vi "FTW-JSON-SetFlags-Encoding.vi"(0 "JSON Object":refnum<class "FTW-JSON.lvclass">, 5 "Indent Spaces":i32=4, 7 "Escape Unicode":bool=TRUE, 9 "Sort Keys":bool, 11 "error in":errorcluster, 12 "Floating Point Significant Digits":i32=16) -> (4 "JSON Object out":refnum<class "FTW-JSON.lvclass">, 15 "error out":errorcluster)   [LabVIEW 2013, in "FTW-JSON.lvclass"]
uses:
  FTW-JSON.lvclass
  FTW-JSON.lvclass/FTW-JSON.ctl
panel:
  # "Inputs"
  # "Outputs"
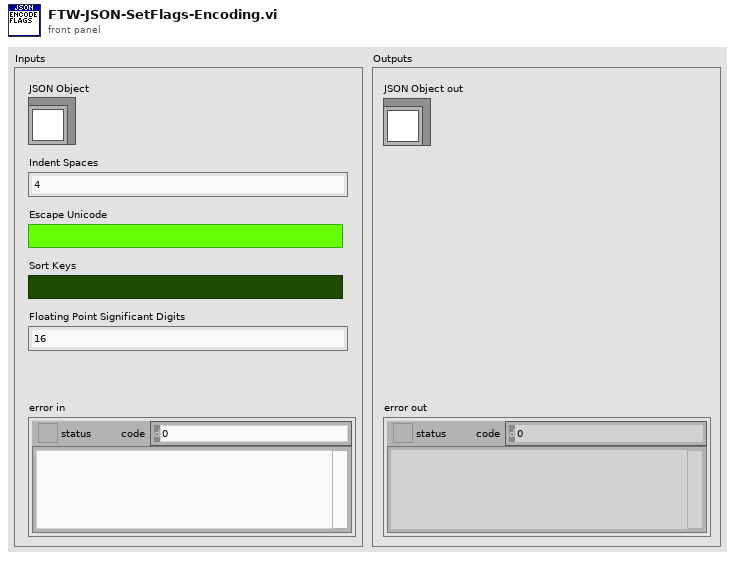
[diagram p1: front panel]
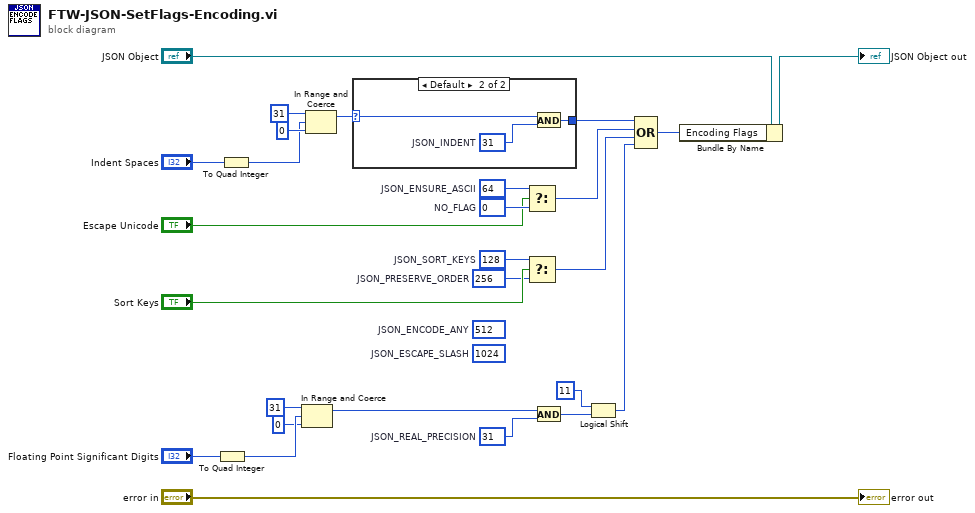
[diagram p0: block diagram]
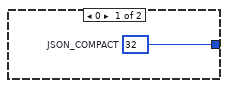
[diagram p2: hidden frame]
diagram:
  w9 = i64 31  # JSON_REAL_PRECISION
  w12 = i64 0  # NO_FLAG
  (unwired) i64 1024  # JSON_ESCAPE_SLASH
  (unwired) i64 512  # JSON_ENCODE_ANY
  w16 = i64 256  # JSON_PRESERVE_ORDER
  w17 = i64 128  # JSON_SORT_KEYS
  w13 = i64 64  # JSON_ENSURE_ASCII
  n1 = To Quad Integer(1:"Floating Point Significant Digits") -> (0:w6:i64)
  n2 = To Quad Integer(1:"Indent Spaces") -> (0:w14:i64)
  n3 = In Range and Coerce(upper limit=i64 31, x=w6, lower limit=i64 0) -> (coerced(x)=w2:i64)  [unwired: 1 out]
  n4 = In Range and Coerce(upper limit=i64 31, x=w14, lower limit=i64 0) -> (coerced(x)=w23:i64)  [unwired: 1 out]
  n5 = case shown="Default" w23 {
    selector: w23 -> [_ w29]
    tunnel: [w28 w30] -> w20
    frame 0 {
      w28 = i64 32  # JSON_COMPACT
    }
    frame Default {
      w31 = i64 31  # JSON_INDENT
      n6 = And(x=w29, y=w31) -> (x .and. y?=w30:i64)
    }
  }
  n7 = Select(t=w13, s="Escape Unicode", f=w12) -> (s? t:f=w10:i64)
  n8 = Select(t=w17, s="Sort Keys", f=w16) -> (s? t:f=w15:i64)
  n9 = And(x=w2, y=w9) -> (x .and. y?=w8:i64)
  n10 = Logical Shift(y=i16 11, x=w8) -> (x << y=w1:i64)
  n11 = Compound Arithmetic op=OR(w20, w10, w15, w1) -> (w19:i64)
  n12 = Bundle By Name(cluster="JSON Object", "Encoding Flags"=w19) -> (→"JSON Object out":refnum<class "FTW-JSON.lvclass">)
  "error out" <- "error in"
